vi "ULx Read (Digital Wfm 1Chan 1Samp).vi"(0 "task in":refnum<k24>, 9 "timeout":dbl=10.0 format="%_4g", 11 "error in":errorcluster) -> (4 "task out":refnum<k24>, 6 "data":digitalwaveform(waveform), 15 "error out":errorcluster)   [LabVIEW 2020]
doc: "Reads a digital waveform that contains a single sample from a task that contains a single digital input channel."
uses:
  C:/Users/William/Documents/LV 2020 builds/LeaktestDAQ/Source-v33/ULx_LV.dll
  ULx_LV.dll
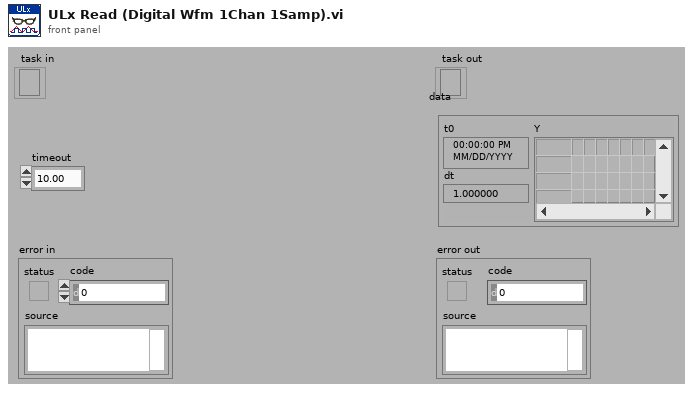
[diagram p1: front panel]
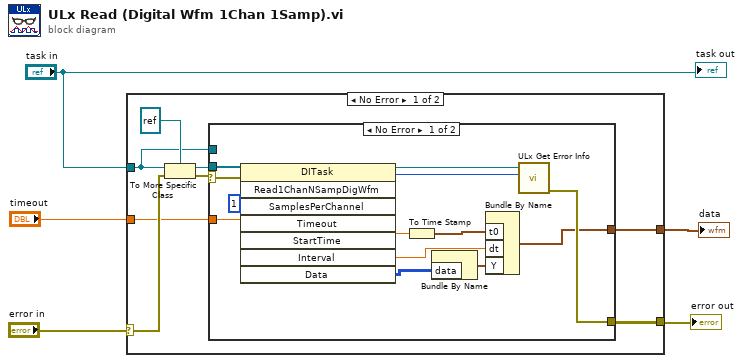
[diagram p0: block diagram]
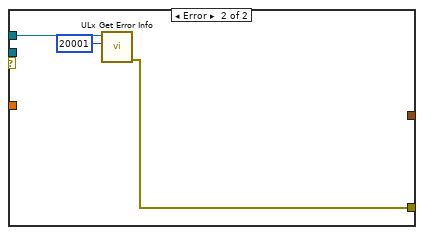
[diagram p2: hidden frame]
diagram:
  n1 = case shown="No Error" "error in" {
    selector: "error in" -> [w13 w30]
    tunnel: "task in" -> [w6 _]
    tunnel: "timeout" -> [w9 _]
    tunnel: [w8 w30] -> w3
    tunnel: [w7 _] -> w1
    frame No Error {
      n2 = To More Specific Class(target class=refnum<k24> refnum, reference=w6, error in=w13) -> (specific class reference=w10:refnum<k24>, error out=w11:errorcluster)
      n3 = case shown="No Error" w11 {
        selector: w11 -> [w25 _]
        tunnel: w10 -> [w26 _]
        tunnel: w9 -> [w16 _]
        tunnel: [w23 w27] -> w8
        tunnel: [w20 _] -> w7
        tunnel: w6 -> [_ w29]
        frame No Error {
          n4 = invoke class="DITask" method="Read1ChanNSampDigWfm"(reference=w26, error in=w25, "SamplesPerChannel"=1, "Timeout"=w16) -> (reference out=w24:refnum<k24>, "Read1ChanNSampDigWfm"=w14:i32, "StartTime"=w17:dbl, "Interval"=w18:dbl, "Data"=w19:u8[][])  [unwired: 4 in, 3 out]
          n5 = To Time Stamp(1:w17) -> (0:w22:timestamp)
          n6 = Bundle By Name("data"=w19) -> (w21:digitaldata)  [unwired: 1 in]
          n7 = Bundle By Name("t0"=w22, "dt"=w18, "Y"=w21) -> (w20:digitalwaveform)  [unwired: 1 in]
          n8 = call "ULx Get Error Info.vi"("ErrorCode"=w14, "task in"=w24) -> ("error out"=w23:errorcluster)  [unwired: 9 in]
        }
        frame Error {
          n9 = call "ULx Get Error Info.vi"("ErrorCode"=20001, "task in"=w29) -> ("error out"=w27:errorcluster)  [unwired: 9 in]
        }
      }
    }
    frame Error {
    }
  }
  "error out" <- w3
  "data" <- w1
  "task out" <- "task in"
